vi "AddChain.vi"(8 "Error In":errorcluster, 10 "Handler":refnum<class "IHandler.lvclass">, 11 "reference in":refnum<class "BaseHandler.lvclass">) -> (0 "Error Out":errorcluster, 3 "reference out":refnum<class "BaseHandler.lvclass">)   [LabVIEW 2020, in "BaseHandler.lvclass"]
uses:
  BaseHandler.lvclass
  IHandler_interface/IHandler.lvclass
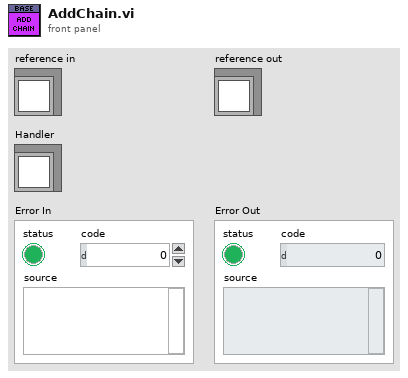
[diagram p1: front panel]
types:
  T1 = typedef "BaseHandler.lvclass/ObjectAttributes.ctl" = cluster{"_nextInLine":refnum<class "IHandler.lvclass">}
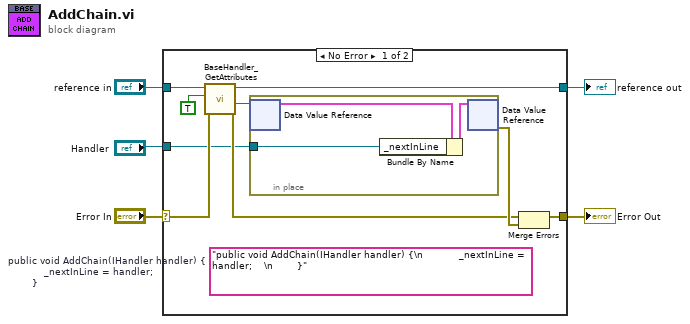
[diagram p0: block diagram]
diagram:
  n1 = case shown="No Error" "Error In" {
    selector: "Error In" -> [w13 w19]
    tunnel: [w10 w19] -> w4
    tunnel: [w11 w18] -> w2
    tunnel: "reference in" -> [w14 w18]
    tunnel: "Handler" -> [w6 _]
    frame No Error {
      (unwired) "public void AddChain(IHandler handler) {\n            _nextInLine = handler;    \n        }"  # public void AddChain(IHandler handler) {             _nextInLine = handler;             }
      n2 = call "BaseHandler_GetAttributes.vi"("error in (no error)"=w13, "OnlyGetDvrReference(False)"=TRUE, "reference in"=w14) -> ("error out"=w8:errorcluster, "DataRef"=w9:refnum<data-value>, "reference out"=w11:refnum<class "BaseHandler.lvclass">)  [unwired: 5 in, 1 out]
      n3 = in-place {
        in-place-border: w6 -> [w15]
        n4 = in-place-dvr #1(w9) -> (w16:T1)  [unwired: 1 out]
        n5 = Bundle By Name(cluster=w16, "_nextInLine"=w15) -> (w17:T1)
        n6 = in-place-dvr #1(w17) -> (w12:errorcluster)  [unwired: 1 out]
      }
      n7 = Merge Errors(w8, w12) -> (w10:errorcluster)
    }
    frame Error {
    }
  }
  "Error Out" <- w4
  "reference out" <- w2
